vi "rqcBob Configure Ramdom Number Generator.vi"(8 "error in":errorcluster, 10 "rqcBob rndGen.parameters":T1={"value type"=enum."constant", "constant"=0, "num of levels"=0, "levels values"=[0, 0, 0, 0]}, 11 "FPGA reference in":refnum<k20>) -> (0 "error out":errorcluster, 3 "FPGA reference out":refnum<k20>)   [LabVIEW 2018]
uses:
  Shared/Shared FPGA Lib/Shared Logic/Custom Controls/rqc Random Generator.parameters.ctl
  Shared/Shared FPGA Lib/Shared Logic/Custom Controls/rqc Random Generator.value type.ctl
  <vilib>/Utility/error.llb/Error Cluster From Error Code.vi
  <vilib>/rvi/errors/niLvFpgaAdjustHostInterfaceError.vi
  <vilib>/rvi/interface/nirviReadWriteControl/nirviReadWriteControl.xnode
  NiFpgaLv.dll
  <vilib>/rvi/interface/Simulation/niFpgaSimulationCallBeginRW.vi
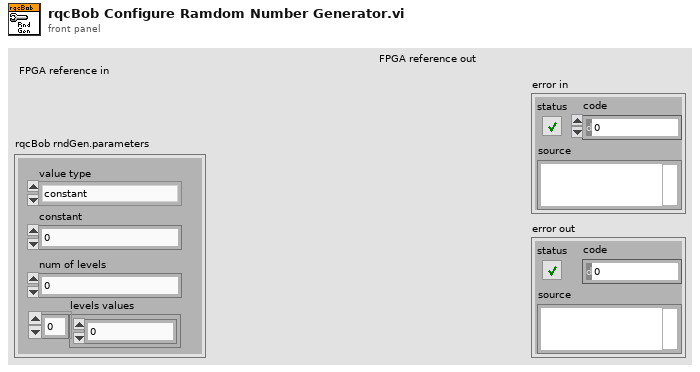
[diagram p1: front panel]
types:
  T1 = typedef "rqc Random Generator.parameters.ctl" = cluster{"value type":T2, "constant":u16, "num of levels":u16, "levels values":u16[]}
  T2 = typedef "rqc Random Generator.value type.ctl" = enum16{"random value", "constant"}
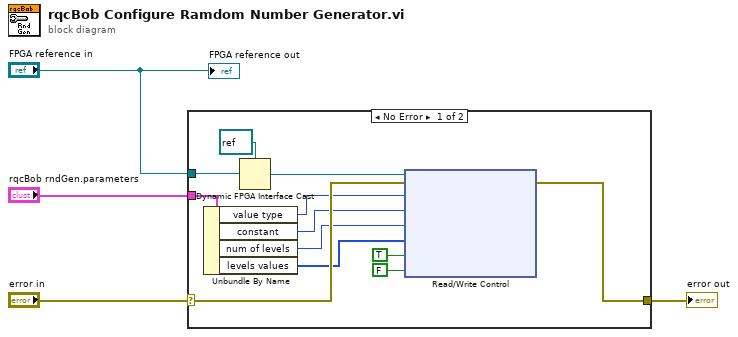
[diagram p0: block diagram]
diagram:
  n1 = case shown="No Error" "error in" {
    selector: "error in" -> [w16 w17]
    tunnel: [w15 w17] -> w2
    tunnel: "FPGA reference in" -> [w13 _]
    tunnel: "rqcBob rndGen.parameters" -> [w9 _]
    frame No Error {
      n2 = Unbundle By Name(w9) -> ("value type"=w8:T2, "constant"=w7:u16, "num of levels"=w6:u16, "levels values"=w5:u16[])
      n3 = Dynamic FPGA Interface Cast(Session In=refnum<k20> refnum ("FPGA Interface"), Type=w13) -> (Session Out=w12:refnum<k20>)
      n4 = xnode "Read/Write Control"("FPGA VI Reference In"=w12, "error in"=w16, "rndGen.value type"=w8, "rndGen.constant"=w7, "rndGen.num of levels"=w6, "rndGen.levels values"=w5, "rndGen.reset"=TRUE, "rndGen.reset"=FALSE) -> ("error out"=w15:errorcluster)  [unwired: 1 out]
    }
    frame Error {
    }
  }
  "error out" <- w2
  "FPGA reference out" <- "FPGA reference in"
